vi "Get Data In.vi"(8 "error in (no error)":errorcluster) -> (0 "error out":errorcluster, 3 "DataIn":T1)   [LabVIEW 2017]
uses:
  TypeDefs/dataIn.ctl
  FGVs/TypeDefs/DataFGVControl.ctl
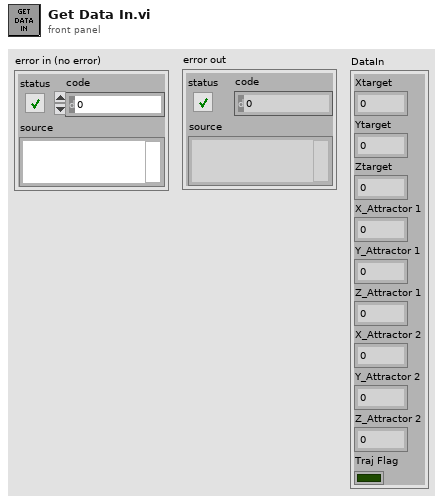
[diagram p1: front panel]
types:
  T1 = typedef "dataIn.ctl" = cluster{"Xtarget":dbl, "Ytarget":dbl, "Ztarget":dbl, "X_Attractor 1":dbl, "Y_Attractor 1":dbl, "Z_Attractor 1":dbl, "X_Attractor 2":dbl, "Y_Attractor 2":dbl, "Z_Attractor 2":dbl, "Traj Flag":bool}
  T2 = typedef "DataFGVControl.ctl" = enum16{"Set Data", "Get Data"}
  T3 = typedef "allData.ctl" = cluster{"DataOut":T4, "DataIn":T1}
  T4 = typedef "dataOut.ctl" = cluster{"Xpos":dbl, "Ypos":dbl, "Zpos":dbl, "Fx":dbl, "Fy":dbl, "Fz":dbl, "Encoder1":i32, "Encoder2":i32, "Pot1":dbl, "Pot2":dbl, "currentTime":timestamp}
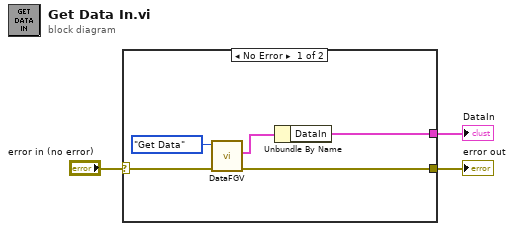
[diagram p0: block diagram]
diagram:
  n1 = case shown="No Error" "error in (no error)" {
    selector: "error in (no error)" -> [w8 w9]
    tunnel: [w7 w9] -> w2
    tunnel: [w4 _] -> w1
    frame No Error {
      n2 = call "DataFGV.vi"("error in (no error)"=w8, "Command"=DataFGVControl."Get Data") -> ("error out"=w7:errorcluster, "AllData out"=w5:T3)  [unwired: 8 in]
      n3 = Unbundle By Name(w5) -> ("DataIn"=w4:T1)
    }
    frame Error {
    }
  }
  "error out" <- w2
  "DataIn" <- w1
